vi "take_picture_pymba (SubVI).vi"(0 "fil path":path=path "C:/Data/20170612/nextday/bead1", 3 "img_cluster":cluster{"Take Pic?":bool}) -> ()   [LabVIEW 2014]
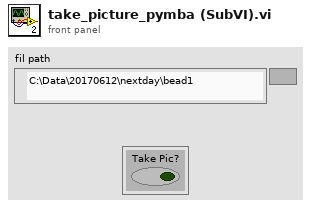
[diagram p1: front panel]
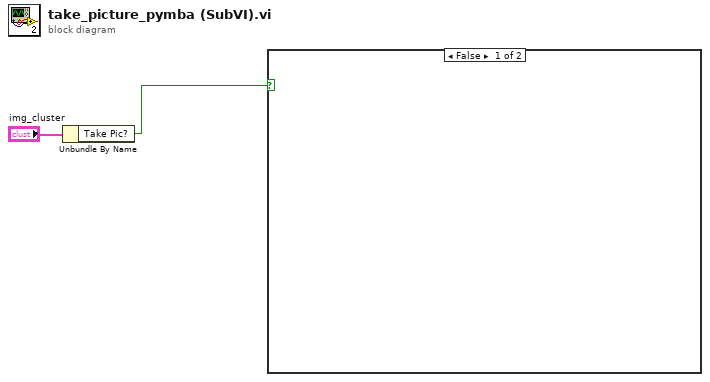
[diagram p0: block diagram]
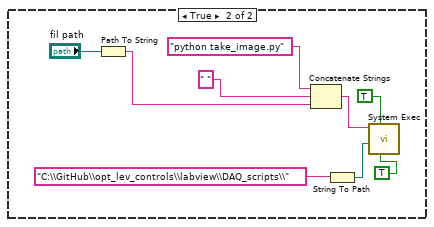
[diagram p2: hidden frame]
diagram:
  n1 = Unbundle By Name("img_cluster") -> ("Take Pic?"=w1:bool)
  n2 = case shown="False" w1 {
    frame False {
    }
    frame True {
      n3 = Path To String(path="fil path") -> (string=w3:string)
      n4 = Concatenate Strings("python take_image.py", " ", w3) -> (w11:string)
      n5 = String To Path(string="C:\\GitHub\\opt_lev_controls\\labview\\DAQ_scripts\\") -> (path=w9:path)
      n6 = call <vilib>:"System Exec.vi"("run minimized? (F)"=TRUE, "wait until completion? (T)"=TRUE, "working directory"=w9, "command line"=w11) -> ()  [unwired: 4 in, 4 out]
    }
  }
